vi "Shutdown.vi"(8 "error in (no error)":errorcluster, 11 "SessionHandler in":refnum<class "SessionHandler.lvclass">) -> ()   [LabVIEW 2019, in "Network Sink.lvlib" / "SessionHandler.lvclass"]
uses:
  <vilib>/gpm_packages/@cs/event-logger/Source/Network Sink/SessionHandler/SessionHandler.lvclass
  <vilib>/gpm_packages/@cs/event-logger/Source/Composed Log/Types/Log Level.ctl
  <vilib>/gpm_packages/@cs/event-logger/Source/Network Sink/SessionHandler/SessionHandler.lvclass/SessionHandler.ctl
  <vilib>/gpm_packages/@cs/Network-Sink/Source/Network Interface/Network Interface/Network Interface.lvclass
  <vilib>/gpm_packages/@cs/event-logger/Source/Composed Log/Composed Log.lvlib
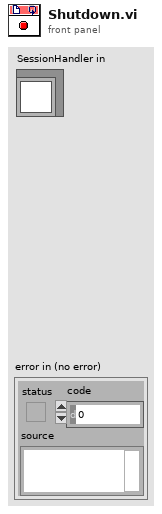
[diagram p1: front panel]
types:
  T1 = typedef "Composed Log.lvlib/Log Level.ctl" = enum16{"Debug", "Info", "Warning", "Error", "Critical"}
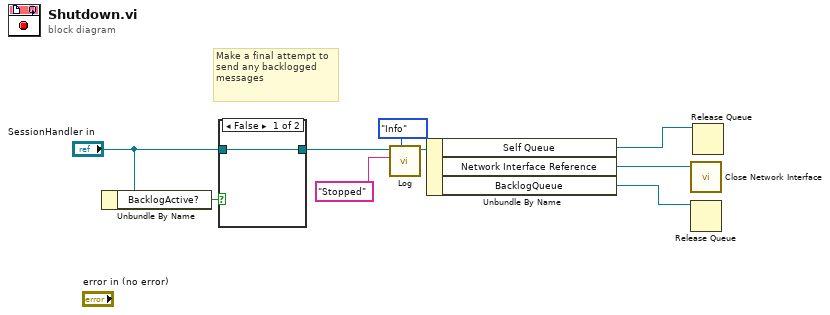
[diagram p0: block diagram]
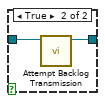
[diagram p2: hidden frame]
diagram:
  # "Make a final attempt to send any backlogged messages"
  n1 = Unbundle By Name("SessionHandler in") -> ("BacklogActive?"=w1:bool)
  n2 = case shown="False" w1 {
    tunnel: [w10 w12] -> w6
    tunnel: "SessionHandler in" -> [w10 w11]
    frame False {
    }
    frame True {
      n3 = call <vilib>:"Attempt Backlog Transmission.vi"("SessionHandler in"=w11) -> ("SessionHandler out"=w12:refnum<class "SessionHandler.lvclass">)  [unwired: 9 in, 1 out]
    }
  }
  n4 = call <vilib>:"Log.vi"("Event Level"=Log_Level."Info", "Data To Log"="Stopped", "SessionHandler in"=w6) -> ("SessionHandler out"=w5:refnum<class "SessionHandler.lvclass">)  [unwired: 7 in, 1 out]
  n5 = Unbundle By Name(w5) -> ("Self Queue"=w8:refnum<queue>, "Network Interface Reference"=w9:refnum<data-value>, "BacklogQueue"=w7:refnum<queue>)
  n6 = call <vilib>:"Close Network Interface.vi"("Network Interface"=w9) -> ()  [unwired: 10 in, 1 out]
  n7 = Release Queue(queue=w7) -> ()  [unwired: 2 in, 3 out]
  n8 = Release Queue(queue=w8) -> ()  [unwired: 2 in, 3 out]
